vi "Clousure.vi"(8 "error in (no error)":errorcluster, 11 "ProductA":refnum<class "ProductA.lvclass">) -> (0 "error out":errorcluster, 3 "ProductA":refnum<class "ProductA.lvclass">)   [LabVIEW 2020, in "FactoryMethod.lvlib" / "FactoryMethodLazyEvaluation.lvlib" / "ProductA.lvclass"]
uses:
  ProductA.lvclass
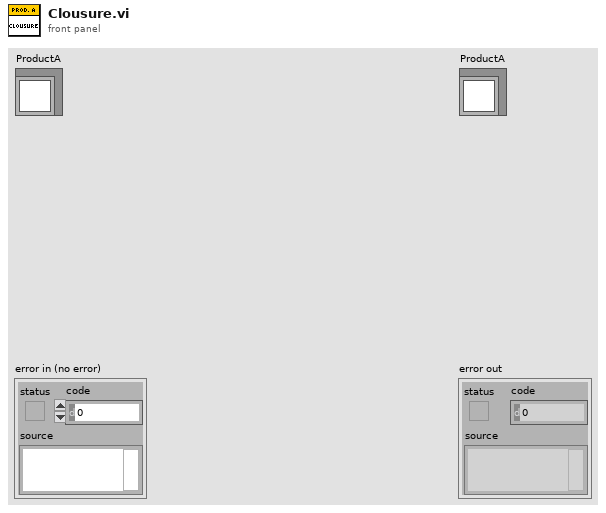
[diagram p1: front panel]
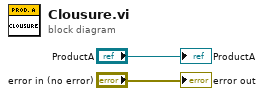
[diagram p0: block diagram]
diagram:
  "error out" <- "error in (no error)"
  "ProductA" <- "ProductA"
